vi "New Subscription Request.vi"(8 "Transport":refnum<class "ITransport.lvclass">, 9 "Unique Subscriber ID":string, 10 "Type":variant, 11 "Topic Name":string) -> (3 "SubscriptionRequest out":refnum<class "SubscriptionRequest.lvclass">)   [LabVIEW 2015, in "IMediator.lvlib" / "SubscriptionRequest.lvclass"]
uses:
  SubscriptionRequest.lvclass
  ITransport/ITransport.lvclass
  SubscriptionRequest.lvclass/SubscriptionRequest.ctl
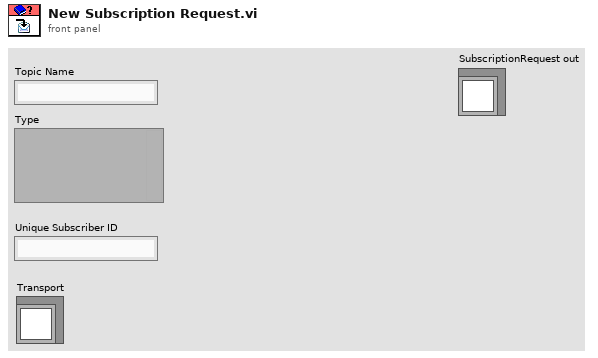
[diagram p1: front panel]
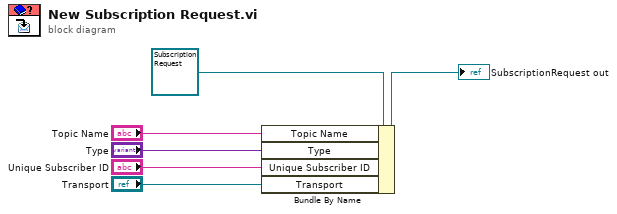
[diagram p0: block diagram]
diagram:
  n1 = Bundle By Name(cluster=refnum<class "SubscriptionRequest.lvclass"> refnum ("SubscriptionRequest in"), "Topic Name"="Topic Name", "Type"="Type", "Unique Subscriber ID"="Unique Subscriber ID", "Transport"="Transport") -> (→"SubscriptionRequest out":refnum<class "SubscriptionRequest.lvclass">)
